vi "Actor Core.vi"(8 "error in":errorcluster, 11 "Python Protocol":refnum<class "Python Protocol.lvclass">) -> (0 "error out":errorcluster, 3 "Actor out":refnum<class "Actor.lvclass">)   [LabVIEW 2012, in "Python Protocol Actor.lvlib" / "Python Protocol.lvclass"]
doc: "This is Actor Core.vi, the main message handling loop for Actors. An actor usually just sits in this loop and processes messages as they arrive. Any error returned by the message Do.vi call will stop the loop, with error code 43 as the canonical signal to stop with no error sent to caller. Descendants may override that in Handle Error.vi."
uses:
  Python Protocol.lvclass
  <vilib>/ActorFramework/Actor/Actor.lvclass
  Python Protocol.lvclass/Python Protocol.ctl
  <vilib>/ActorFramework/Actor/Actor.lvclass/Actor.ctl
  <vilib>/ActorFramework/Message Enqueuer/Message Enqueuer.lvclass/Message Enqueuer.ctl
  Python Protocol Messages/Change Status Msg/Change Status Msg.lvclass/Change Status Msg.ctl
  Read DVR.vi
  Write Start Time.vi
  Write Ring Refnum.vi
  Write Open.vi
  Write Save.vi
  Write Refresh.vi
  Write State.vi
  Write New.vi
  Write Path.vi
  Write Code.vi
  Write Compiler.vi
  Write VI Refnum.vi
  <vilib>/ActorFramework/Message Enqueuer/Init from Existing Queue.vi
  <vilib>/ActorFramework/Message Enqueuer/Enqueue.vi
  <vilib>/ActorFramework/Message Priority Queue/Priority Enqueue.vi
  <vilib>/ActorFramework/Message Enqueuer/Message Enqueuer.lvclass
  <vilib>/ActorFramework/Stop Msg/Stop Msg.lvclass
  Python Protocol Messages/Run Protocol Msg/Run Protocol Msg.lvclass
  Python Protocol Messages/New Protocol Msg/New Protocol Msg.lvclass
  Python Protocol Messages/Open Protocol Msg/Open Protocol Msg.lvclass
  Python Protocol Messages/Save Protocol Msg/Save Protocol Msg.lvclass
  Python Protocol Messages/Compile Protocol Msg/Compile Protocol Msg.lvclass
  Python Protocol Messages/Change Status Msg/Change Status Msg.lvclass
  Python Protocol Messages/Insert Variable Msg/Insert Variable Msg.lvclass
panel:
  in  "stop signal":bool
  in  "Menu Ring":u16(ring) items=["fgfdgdfgdfg", ""]
  in  "Radio Buttons":T1(radio)=enum."Media Stop Button"
  in  "Open Button":bool
  in  "New Button":bool
  in  "Refresh Button":bool
  in  "Save Button":bool
  out "File Path Control":path
  in  "Code":string
  out "Compiler":string
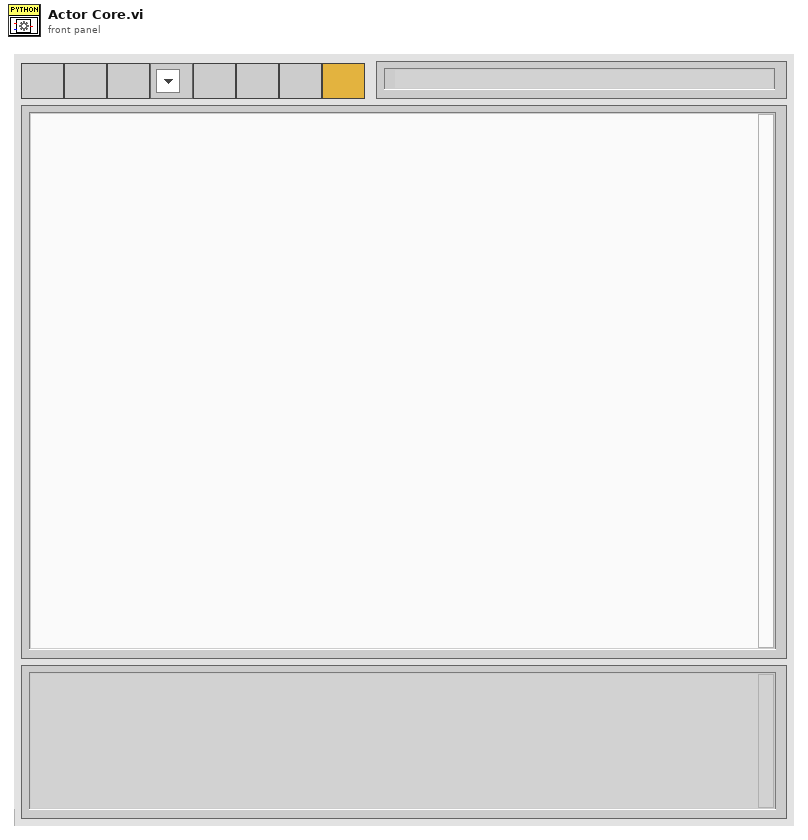
[diagram p1: front panel]
types:
  T1 = enum32{"Pause Button", "Play Button", "Media Stop Button"}
  T2 = cluster{"Name":string, "Value":dbl, "Setpoint":dbl, "Output":dbl}[]
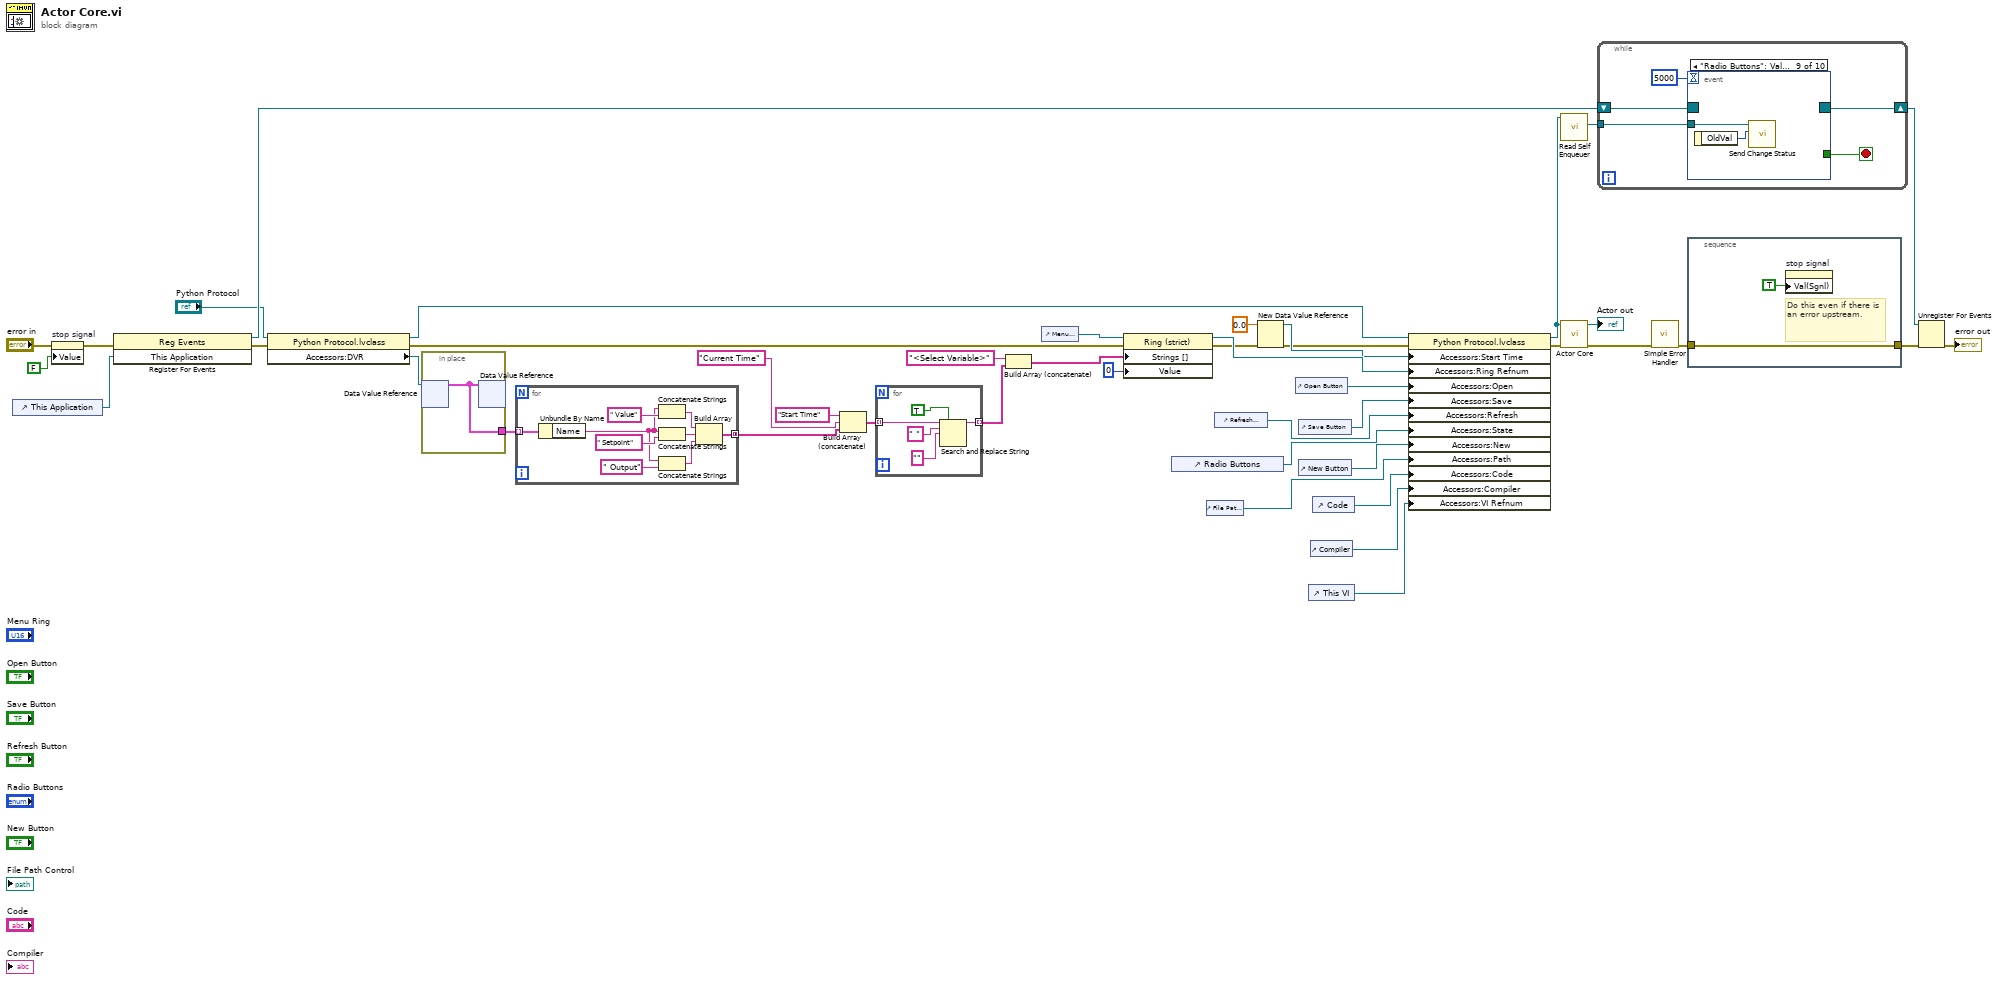
[diagram p0: block diagram]
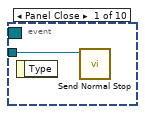
[diagram p2: hidden frame]
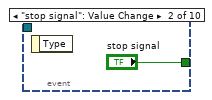
[diagram p3: hidden frame]
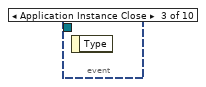
[diagram p4: hidden frame]
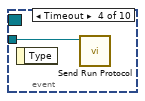
[diagram p5: hidden frame]
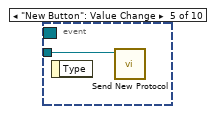
[diagram p6: hidden frame]
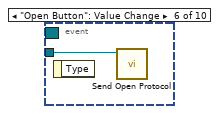
[diagram p7: hidden frame]
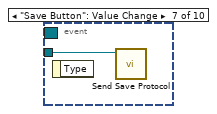
[diagram p8: hidden frame]
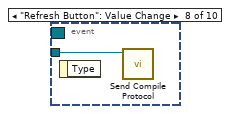
[diagram p9: hidden frame]
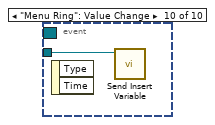
[diagram p10: hidden frame]
diagram:
  n1 = control-ref of="This Application"() -> (w35:refnum<vi>)
  n2 = property on="stop signal" class="Bool (strict)"(error in="error in", "Value"=FALSE ("stop")) -> (error out=w36:errorcluster)  [unwired: 1 in, 1 out]
  n3 = register-events(error in=w36, w35) -> (reference out=w39:refnum<event-registration>, error out=w12:errorcluster)  [unwired: 1 in]
  n4 = property class="Python Protocol.lvclass"(reference="Python Protocol", error in=w12) -> (reference out=w18:refnum<class "Python Protocol.lvclass">, error out=w13:errorcluster, "Accessors:DVR"=w14:refnum<data-value>)
  n5 = in-place {
    in-place-border: [w44] -> w17
    n6 = in-place-dvr #1(w14) -> (w44:T2)  [unwired: 1 out]
    n7 = in-place-dvr #1(w44) -> ()  [unwired: 2 out]
  }
  n8 = for {
    tunnel: w17 -> [w53] mode=indexing
    tunnel: [w45] -> w16 mode=concatenating
    n9 = Unbundle By Name(w53) -> ("Name"=w46:string)
    n10 = Concatenate Strings(w46, " Value" ("string")) -> (w49:string)
    n11 = Concatenate Strings(w46, " Setpoint" ("string")) -> (w48:string)
    n12 = Concatenate Strings(w46, " Output" ("string")) -> (w47:string)
    n13 = Build Array(w49, w48, w47) -> (w45:string[])
  }
  n14 = Build Array (concatenate)("Start Time" ("element"), "Current Time", w16) -> (w15:string[])
  n15 = for {
    tunnel: w15 -> [w58] mode=indexing
    tunnel: [w54] -> w10 mode=indexing
    n16 = Search and Replace String(replace all?=TRUE ("replace all? (F)"), input string=w58, search string=" ", replace string="" ("replace string (\"\")")) -> (result string=w54:string)  [unwired: 4 in, 3 out]
  }
  n17 = Build Array (concatenate)("<Select Variable>", w10) -> (w9:string[])
  n18 = control-ref of="Menu Ring"() -> (w20:refnum<vi>)
  n19 = property class="Ring (strict)"(reference=w20, error in=w13, "Strings []"=w9, "Value"=u16 0) -> (reference out=w6:refnum<vi>, error out=w3:errorcluster)
  n20 = control-ref of="Radio Buttons"() -> (w28:refnum<vi>)
  n21 = control-ref of="File Path Control"() -> (w26:refnum<vi>)
  n22 = control-ref of="Refresh Button"() -> (w29:refnum<vi>)
  n23 = New Data Value Reference(data value=0.0, error in=w3) -> (data value reference=w5:refnum<data-value>, error out=w4:errorcluster)
  n24 = control-ref of="Open Button"() -> (w21:refnum<vi>)
  n25 = control-ref of="Save Button"() -> (w30:refnum<vi>)
  n26 = control-ref of="New Button"() -> (w27:refnum<vi>)
  n27 = control-ref of="This VI"() -> (w23:refnum<vi>)
  n28 = control-ref of="Compiler"() -> (w24:refnum<vi>)
  n29 = control-ref of="Code"() -> (w25:refnum<vi>)
  n30 = property class="Python Protocol.lvclass"(reference=w18, error in=w4, "Accessors:Start Time"=w5, "Accessors:Ring Refnum"=w6, "Accessors:Open"=w21, "Accessors:Save"=w30, "Accessors:Refresh"=w29, "Accessors:State"=w28, "Accessors:New"=w27, "Accessors:Path"=w26, "Accessors:Code"=w25, "Accessors:Compiler"=w24, "Accessors:VI Refnum"=w23) -> (reference out=w22:refnum<class "Python Protocol.lvclass">, error out=w34:errorcluster)
  n31 = call <vilib>:"Read Self Enqueuer.vi"("Actor"=w22) -> ("Self Enqueuer"=w43:refnum<class "Message Enqueuer.lvclass">)  [unwired: 10 in]
  n32 = call-parent "Actor Core.vi"("error in"=w34, "Actor in"=w22) -> ("error out"=w41:errorcluster, "Actor out"=→"Actor out":refnum<class "Actor.lvclass">)  [unwired: 8 in]
  n33 = while {
    tunnel: w43 -> [w63]
    shift-right: [w60] -> w38
    shift-left: w39 -> [w61]
    stop <- w62 stop-if-true
    n34 = event shown="[8] \"Radio Buttons\": Value Change" {
      selector: w61 -> [_ _ _ _ _ _ _ _ _ _]
      dyn-events: [_ _ _ _ _ _ _ _ _ _] -> w60
      timeout: 5000 -> [_ _ _ _ _ _ _ _ _ _]
      tunnel: w63 -> [w64 _ _ w66 w67 w68 w69 w70 w72 w73]
      tunnel: [_ "stop signal" _ _ _ _ _ _ _ _] -> w62
      event Panel Close {
        n35 = event-data() -> ()  [unwired: 1 in, 1 out]
        n36 = call <vilib>:"Send Normal Stop.vi"("Message Enqueuer"=w64) -> ()  [unwired: 10 in, 1 out]
      }
      event "stop signal": Value Change {
        n37 = event-data() -> ()  [unwired: 1 in, 1 out]
      }
      event Application Instance Close {
        n38 = event-data() -> ()  [unwired: 1 in, 1 out]
      }
      event Timeout {
        n39 = event-data() -> ()  [unwired: 1 in, 1 out]
        n40 = call "Send Run Protocol.vi"("Message Enqueuer"=w66) -> ()  [unwired: 9 in, 2 out]
      }
      event "New Button": Value Change {
        n41 = event-data() -> ()  [unwired: 1 in, 1 out]
        n42 = call "Send New Protocol.vi"("Message Enqueuer"=w67) -> ()  [unwired: 9 in, 2 out]
      }
      event "Open Button": Value Change {
        n43 = event-data() -> ()  [unwired: 1 in, 1 out]
        n44 = call "Send Open Protocol.vi"("Message Enqueuer"=w68) -> ()  [unwired: 9 in, 2 out]
      }
      event "Save Button": Value Change {
        n45 = event-data() -> ()  [unwired: 1 in, 1 out]
        n46 = call "Send Save Protocol.vi"("Message Enqueuer"=w69) -> ()  [unwired: 9 in, 2 out]
      }
      event "Refresh Button": Value Change {
        n47 = event-data() -> ()  [unwired: 1 in, 1 out]
        n48 = call "Send Compile Protocol.vi"("Message Enqueuer"=w70) -> ()  [unwired: 9 in, 2 out]
      }
      event "Radio Buttons": Value Change {
        n49 = event-data() -> ("OldVal"=w71:T1)  [unwired: 1 in]
        n50 = call "Send Change Status.vi"("Old Value"=w71, "Message Enqueuer"=w72) -> ()  [unwired: 8 in, 2 out]
      }
      event "Menu Ring": Value Change {
        n51 = event-data() -> ()  [unwired: 1 in, 2 out]
        n52 = call "Send Insert Variable.vi"("Message Enqueuer"=w73) -> ()  [unwired: 9 in, 2 out]
      }
    }
  }
  n53 = call <vilib>:"Simple Error Handler.vi"("error in (no error)"=w41) -> ("error out"=w40:errorcluster)  [unwired: 4 in, 4 out]
  n54 = stacked-sequence {
    tunnel: [w74] -> w37
    tunnel: w40 -> [w74]
    frame #0 {
      # "Do this even if there is an error upstream."
      n55 = property on="stop signal" class="Bool (strict)"("Val(Sgnl)"=TRUE ("stop")) -> ()  [unwired: 2 in, 2 out]
    }
  }
  n56 = Unregister For Events(event registration refnum=w38, error in=w37) -> (error out=→"error out":errorcluster)
